vi "Create MDIF Variable Array.vi"(8 "error in (no error)":errorcluster, 10 "Values":variant, 11 "Name":string) -> (0 "error out":errorcluster, 3 "MDIF Variable":cluster{"Name":string, "Values":refnum<k24>})   [LabVIEW 2023, in "NI_HFNetworkAnalysis.lvlib"]
doc: "Creates a MDIF Variable Array with the specified name and values to be compliant with the array elements of the <b>Independent Variables</b> and <b>Dependent Variables</b> inputs of the <b>Add MDIF Block.vi</b>."
uses:
  NI_HFNetworkAnalysis.lvlib
  C:/srd-semi-rfcal-software/AuxTools/STSRFFixtureCharactUtility/Source/Code Modules/Fixture/Dependencies/HFNetworkAnalysis/Support Files/NACE.Utils.Data.dll
  Support Files/NACE.Utils.Data.dll
  <vilib>/Utility/VariantDataType/VariantType.lvlib
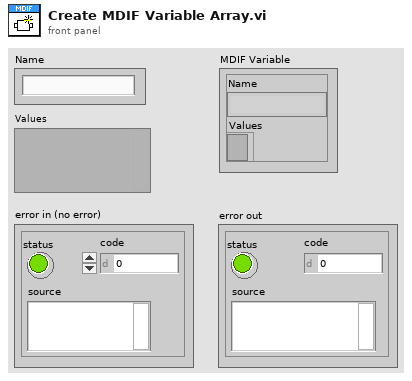
[diagram p1: front panel]
types:
  T1 = typedef "VariantType.lvlib/Type.ctl" = enum8{"Invalid Type", "Void", "I8", "I16", "I32", "I64", "U8", "U16", "U32", "U64", "Single Float", "Double Float", "Extended Float", "Single Complex", "Double Complex", "Extended Complex", "Enum U8", "Enum U16", "Enum U32", "Enum U64", "Single Float With Unit", "Double Float With Unit", "Extended Float With Unit", "Single Complex with Unit", "Double Complex with Unit", "Extended Complex with Unit", "Boolean", "String", "Path", "Picture", "Tag", "Array", "Cluster", "Variant", "LV Variant", "Waveform", "Timestamp", "Digital Waveform", "Digital Data", "ExpressData", "Refnum", "External Data", "VI", "Poly VI", "LabVIEW Class Instance", "Fixed Point"}
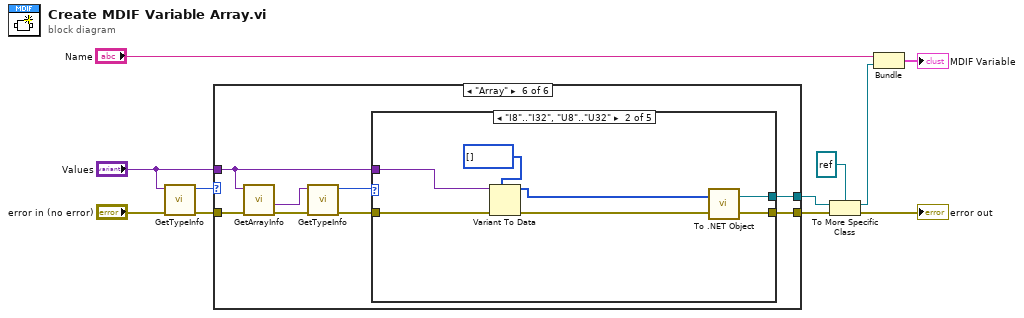
[diagram p0: block diagram]
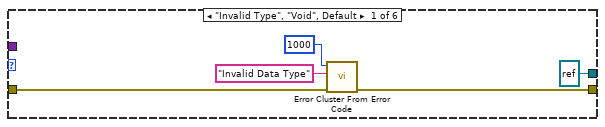
[diagram p2: hidden frame]
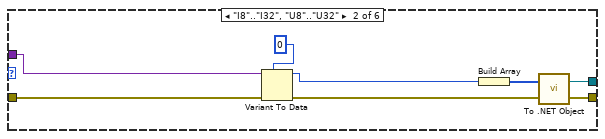
[diagram p3: hidden frame]
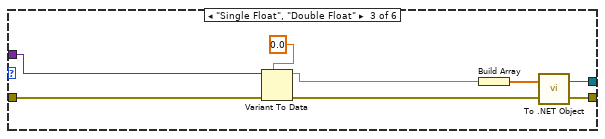
[diagram p4: hidden frame]
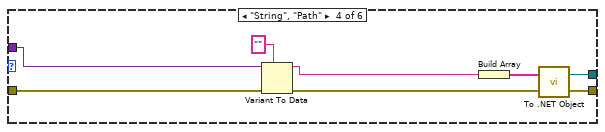
[diagram p5: hidden frame]
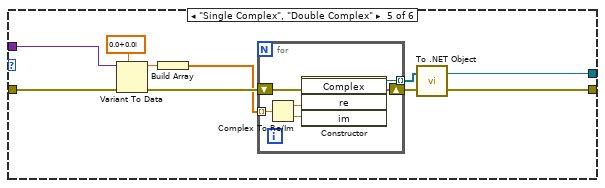
[diagram p6: hidden frame]
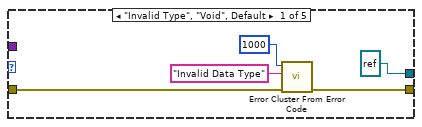
[diagram p7: hidden frame]
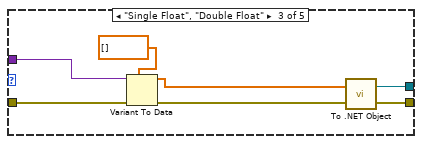
[diagram p8: hidden frame]
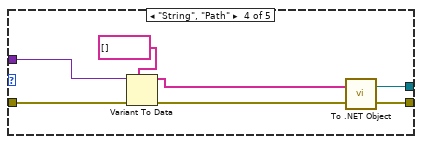
[diagram p9: hidden frame]
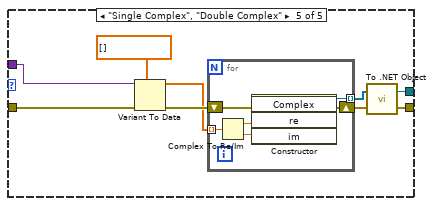
[diagram p10: hidden frame]
diagram:
  n1 = call <vilib>:"GetTypeInfo.vi"("error in (no error)"="error in (no error)", "Variant"="Values") -> ("error out"=w10:errorcluster, "Type Enum"=w11:T1)  [unwired: 5 in, 3 out]
  n2 = case shown="\"Array\"" w11 {
    tunnel: "Values" -> [_ w19 w27 w35 w50 w59]
    tunnel: w10 -> [w14 w21 w29 w37 w47 w64]
    tunnel: [refnum<k24> refnum (".NET object") w23 w31 w39 w42 w58] -> w8
    tunnel: [w13 w24 w32 w40 w41 w57] -> w7
    frame "Invalid Type", "Void", Default {
      n3 = call <vilib>:"Error Cluster From Error Code.vi"("error in (no error)"=w14, "error message (\"\")"="Invalid Data Type" ("error message (\"\")"), "error code (0)"=1000) -> ("error out"=w13:errorcluster)  [unwired: 6 in]
    }
    frame "I8".."I32", "U8".."U32" {
      n4 = Variant To Data(error in=w21, type=0, Variant=w19) -> (data=w18:i32, error out=w20:errorcluster)
      n5 = Build Array(w18) -> (w22:i32[])
      n6 = call <vilib>:"To .NET Object.vi"("error in (no error)"=w20, "anything"=w22) -> ("error out"=w24:errorcluster, ".NET object"=w23:refnum<k24>)
    }
    frame "Single Float", "Double Float" {
      n7 = Variant To Data(error in=w29, type=0.0, Variant=w27) -> (data=w26:dbl, error out=w28:errorcluster)
      n8 = Build Array(w26) -> (w30:dbl[])
      n9 = call <vilib>:"To .NET Object.vi"("error in (no error)"=w28, "anything"=w30) -> ("error out"=w32:errorcluster, ".NET object"=w31:refnum<k24>)
    }
    frame "String", "Path" {
      n10 = Variant To Data(error in=w37, type="", Variant=w35) -> (data=w34:string, error out=w36:errorcluster)
      n11 = Build Array(w34) -> (w38:string[])
      n12 = call <vilib>:"To .NET Object.vi"("error in (no error)"=w36, "anything"=w38) -> ("error out"=w40:errorcluster, ".NET object"=w39:refnum<k24>)
    }
    frame "Single Complex", "Double Complex" {
      n13 = Variant To Data(error in=w47, type=cdb 0.0+0.0i, Variant=w50) -> (data=w46:cdb, error out=w48:errorcluster)
      n14 = Build Array(w46) -> (w45:cdb[])
      n15 = for {
        tunnel: w45 -> [w53] mode=indexing
        tunnel: [w52] -> w44 mode=indexing
        shift-right: [w51] -> w43
        shift-left: w48 -> [w56]
        n16 = Complex To Re/Im(x + iy=w53) -> (x=w55:dbl, y=w54:dbl)
        n17 = constructor class="Complex"(error in=w56, "re"=w55, "im"=w54) -> (reference out=w52:refnum<k24>, error out=w51:errorcluster)  [unwired: 2 in, 3 out]
      }
      n18 = call <vilib>:"To .NET Object.vi"("error in (no error)"=w43, "anything"=w44) -> ("error out"=w41:errorcluster, ".NET object"=w42:refnum<k24>)
    }
    frame "Array" {
      n19 = call <vilib>:"GetArrayInfo.vi"("error in (no error)"=w64, "Variant"=w59) -> ("error out"=w62:errorcluster, "ArrayElement"=w63:variant)  [unwired: 6 in, 2 out]
      n20 = call <vilib>:"GetTypeInfo.vi"("error in (no error)"=w62, "Variant"=w63) -> ("error out"=w60:errorcluster, "Type Enum"=w61:T1)  [unwired: 5 in, 3 out]
      n21 = case shown="\"I8\"..\"I32\", \"U8\"..\"U32\"" w61 {
        tunnel: w60 -> [w68 w72 w79 w86 w96]
        tunnel: w59 -> [_ w74 w81 w88 w95]
        tunnel: [refnum<k24> refnum (".NET object") w75 w82 w89 w93] -> w58
        tunnel: [w67 w76 w83 w90 w92] -> w57
        frame "Invalid Type", "Void", Default {
          n22 = call <vilib>:"Error Cluster From Error Code.vi"("error in (no error)"=w68, "error message (\"\")"="Invalid Data Type" ("error message (\"\")"), "error code (0)"=1000) -> ("error out"=w67:errorcluster)  [unwired: 6 in]
        }
        frame "I8".."I32", "U8".."U32" {
          n23 = Variant To Data(error in=w72, type=i32[] [], Variant=w74) -> (data=w73:i32[], error out=w71:errorcluster)
          n24 = call <vilib>:"To .NET Object.vi"("error in (no error)"=w71, "anything"=w73) -> ("error out"=w76:errorcluster, ".NET object"=w75:refnum<k24>)
        }
        frame "Single Float", "Double Float" {
          n25 = Variant To Data(error in=w79, type=dbl[] [], Variant=w81) -> (data=w80:dbl[], error out=w78:errorcluster)
          n26 = call <vilib>:"To .NET Object.vi"("error in (no error)"=w78, "anything"=w80) -> ("error out"=w83:errorcluster, ".NET object"=w82:refnum<k24>)
        }
        frame "String", "Path" {
          n27 = Variant To Data(error in=w86, type=string[] [], Variant=w88) -> (data=w87:string[], error out=w85:errorcluster)
          n28 = call <vilib>:"To .NET Object.vi"("error in (no error)"=w85, "anything"=w87) -> ("error out"=w90:errorcluster, ".NET object"=w89:refnum<k24>)
        }
        frame "Single Complex", "Double Complex" {
          n29 = Variant To Data(error in=w96, type=cdb[] [], Variant=w95) -> (data=w94:cdb[], error out=w97:errorcluster)
          n30 = for {
            tunnel: w94 -> [w102] mode=indexing
            tunnel: [w101] -> w98 mode=indexing
            shift-right: [w100] -> w99
            shift-left: w97 -> [w105]
            n31 = Complex To Re/Im(x + iy=w102) -> (x=w104:dbl, y=w103:dbl)
            n32 = constructor class="Complex"(error in=w105, "re"=w104, "im"=w103) -> (reference out=w101:refnum<k24>, error out=w100:errorcluster)  [unwired: 2 in, 3 out]
          }
          n33 = call <vilib>:"To .NET Object.vi"("error in (no error)"=w99, "anything"=w98) -> ("error out"=w92:errorcluster, ".NET object"=w93:refnum<k24>)
        }
      }
    }
  }
  n34 = To More Specific Class(target class=refnum<k24> refnum, reference=w8, error in=w7) -> (specific class reference=w3:refnum<k24>, error out=→"error out":errorcluster)
  n35 = Bundle("Name"="Name", w3) -> (→"MDIF Variable":cluster{"Name":string, refnum<k24>})  [unwired: 1 in]
